vi "HoloPy_get_reconstruction_plane.vi"(8 "error in (no error)":errorcluster, 10 "plane number":u16, 11 "Refnum in":refnum<k35>) -> (0 "error out":errorcluster, 1 "HOLO_array":sgl[][](array[numeric]), 3 "Refnum out":refnum<k35>)   [LabVIEW 2023, in "holoPyTracks.lvlib"]
uses:
  holoPyTracks.lvlib
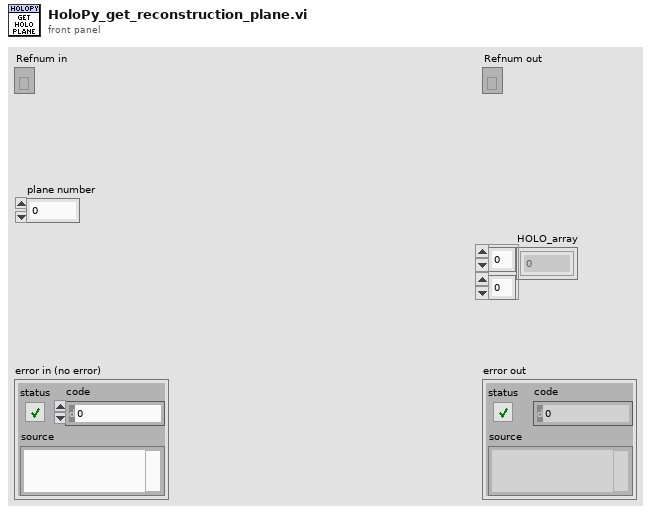
[diagram p1: front panel]
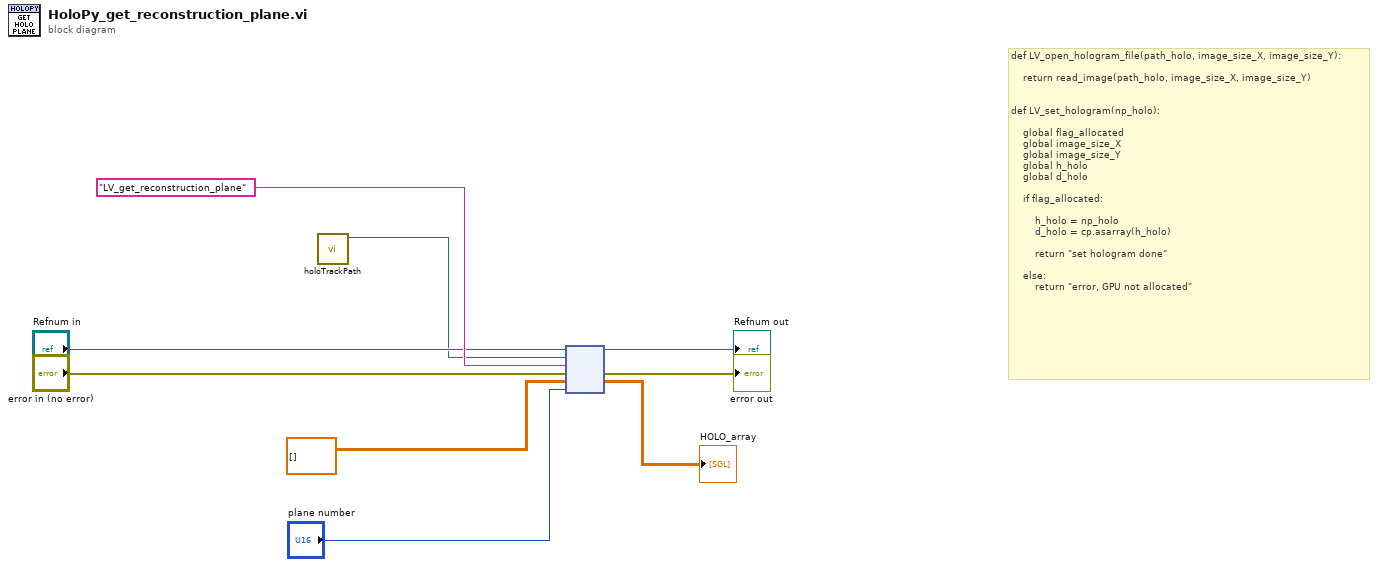
[diagram p0: block diagram]
diagram:
  # "def LV_open_hologram_file(path_holo, image_size_X, image_size_Y):\n\n    return read_image(path_holo, image_size_X, image_size_Y)\n\n\ndef LV_set_hologram(np_holo):\n\n    global flag_allocated\n    global image_size_X \n    global image_size_Y \n    global h_holo\n    global d_holo\n\n    if flag_allocated:\n\n        h_holo = np_holo\n        d_holo = cp.asarray(h_holo)\n\n        return \"set hologram done\"\n    \n    else:\n        return \"error, GPU not allocated\""
  n1 = call "holoTrackPath.vi"() -> ("appended path"=w2:path)  [unwired: 11 in]
  n2 = node("Refnum in", w2, "LV_get_reconstruction_plane" ("function name"), "error in (no error)", sgl[][] [] ("HOLO_array"), "plane number") -> (→"Refnum out":refnum<k35>, →"error out":errorcluster, →"HOLO_array":sgl[][])  [unwired: 1 in, 2 out]
